vi "tag_lens_trigger.vi"() -> (2 "trigger out":bool)   [LabVIEW 2010]
uses:
  <vilib>/eio/EIONode/EIONode.xnode
  <vilib>/rvi/eio/nirviEIOImplementation/nirviEIOImplementation.xnode
  <vilib>/rvi/eio/common/nirviEmuClasses.ctl
  <vilib>/rvi/eio/common/nirviEmuTemplateMethod_noerrors.vi
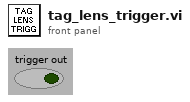
[diagram p1: front panel]
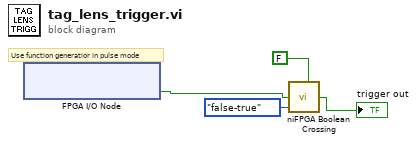
[diagram p0: block diagram]
diagram:
  # "Use function generatior in pulse mode"
  n1 = xnode "FPGA I/O Node"() -> ("Connector0/DIO6"=w2:bool)  [unwired: 1 in, 1 out]
  n2 = call <vilib>:"niFPGA Boolean Crossing.vi"("input"=w2, "direction"=enum8{"either", "false-true", "true-false"}."false-true", "initialize"=FALSE) -> ("crossing"=→"trigger out":bool)  [unwired: 6 in]
